vi "Test_Impression_Etiquette_Carton.vi"() -> ()   [LabVIEW 2020]
uses:
  Modules/Fonction Standard/Fichier ou dossier/Cluster des Chemins.ctl
  Flatprop/Flatprop - Standard/XML/Control/PP Param_3.ctl
panel:
  in  "DIVISION":enum16{"FLATPROP", "MEDIC"}(ring)
  in  "Pieces/carton":u16=25
  in  "Paramètres Produit (PP)":T1={"Numéro T121"="", "Créateur"="", "Date de création"="", "Date de modification"="", "indice produit"="03", "Code Barre fixe"="11210574", "Affiche n° Client [Oui/Non]"="Oui", "Fichier PTV"="", "Nbr de valves / Cartons"="25", "Mélange des lots posiible [Oui/Non] "="Non", "Affiche code barre client [Oui/Non]"="Oui", "Fichier PP valve sur embase"="", "Valve Direct/Compensée [D/C]"="D"} caption="Paramètres produit"
  in  "DATA cmde":T2={"n°article FAS"="12-216C-04521 EQIFIL 417mA 14.4ohm", "n° cmde FAS"="03838/08-01.07.01", "quantité cmde"="100", "ID LIG cmde"="966584", "n° cmde client"="CF-08-0253/2", "nom client"="EMS Electro Medical System", "n° article client"="EL-360", "indice revision client"="03", "société de facturation"="FAS Medic", "langue a utiliser"="FR"}
  in  "error in (no error)":errorcluster caption="entrée d'erreur (pas d'erreur)"
  out "error out":errorcluster caption="sortie d'erreur"
  # "Positionner sur \"MEDIC\"\npour prise en compte indicateur \n\"Pieces/carton\""
  # "Ssi Division \"MEDIC\""
  # "etiquette"
  # "(Lien interchangeable)"
  # "emballage"
  # "emballage"
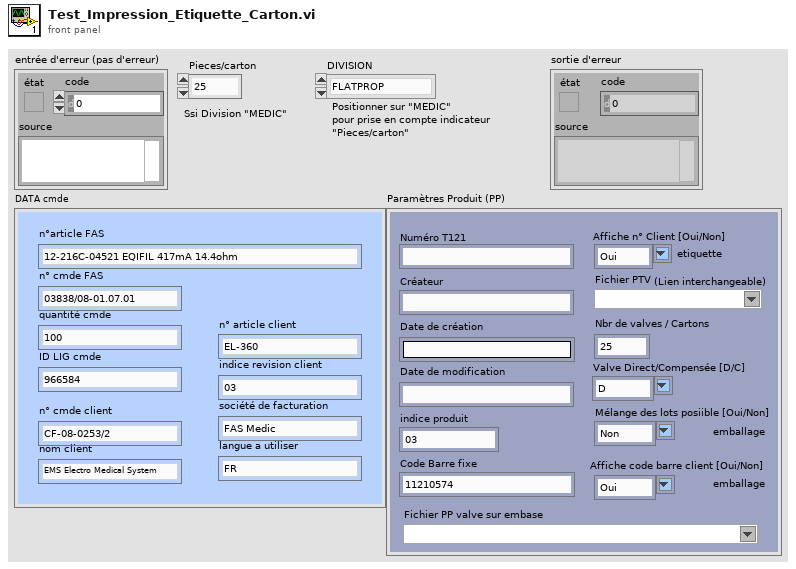
[diagram p1: front panel]
types:
  T1 = typedef "PP Param_3.ctl" = cluster{"Numéro T121":string, "Créateur":string, "Date de création":string, "Date de modification":string, "indice produit":string, "Code Barre fixe":string, "Affiche n° Client [Oui/Non]":string, "Fichier PTV":string, "Nbr de valves / Cartons":string, "Mélange des lots posiible [Oui/Non] ":string, "Affiche code barre client [Oui/Non]":string, "Fichier PP valve sur embase":string, "Valve Direct/Compensée [D/C]":string}
  T2 = typedef "DATA commande.ctl" = cluster{"n°article FAS":string, "n° cmde FAS":string, "quantité cmde":string, "ID LIG cmde":string, "n° cmde client":string, "nom client":string, "n° article client":string, "indice revision client":string, "société de facturation":string, "langue a utiliser":string}
  T3 = enum16{"Sans_imprimante", "Zebra_Medic_emballage2", "Zebra_Medic_2", "Zebra_Medic_1", "Zebra_Flat_emballage"}
  T4 = typedef "Cluster des Chemins.ctl" = cluster{" Admin-réseau ":path, " XML-Réseau":path, " Résultat tests-Réseau":path, " Archive prôbleme-Réseau":path, " Archive Test  Local":path}
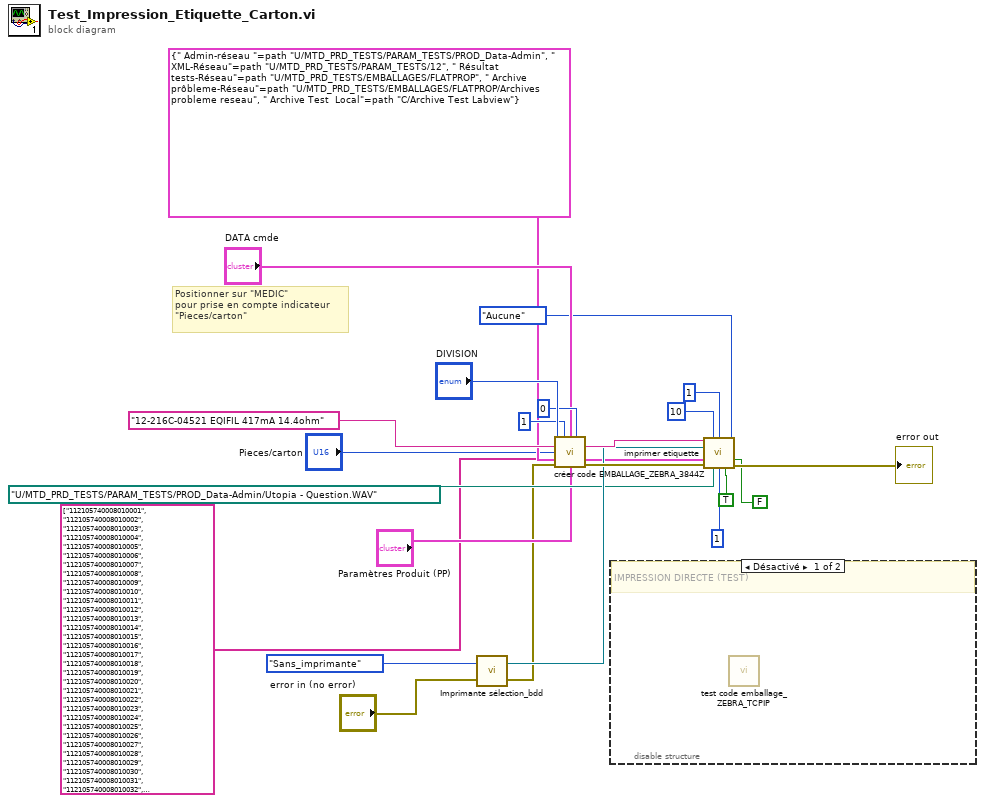
[diagram p0: block diagram]
diagram:
  # "Positionner sur \"MEDIC\"\npour prise en compte indicateur \n\"Pieces/carton\""
  n1 = call "Imprimante sélection_bdd.vi"("entrée d'erreur"="error in (no error)", "Choix imprimante"=T3."Sans_imprimante") -> ("sortie d'erreur"=w2:errorcluster, "Output ressource VISA"=w13:refnum<visa-resource-name>)
  n2 = call "créer code EMBALLAGE_ZEBRA_3844Z.vi"("DIVISION"="DIVISION", "N° carton"=u8 1, "DATA cmde"="DATA cmde", "Nb total cartons"=0, 5:"12-216C-04521 EQIFIL 417mA 14.4ohm" ("article"), 7:"Pieces/carton", "Tableau n° valves"=string[] ["112105740008010001", "112105740008010002", "112105740008010003", "112105740008010004", "112105740008010005", "112105740008010006", "112105740008010007", "112105740008010008", "112105740008010009", "112105740008010010", "112105740008010011", "112105740008010012", "112105740008010013", "112105740008010014", "112105740008010015", "112105740008010016", "112105740008010017", "112105740008010018", "112105740008010019", "112105740008010020", "112105740008010021", "112105740008010022", "112105740008010023", "112105740008010024", "112105740008010025", "112105740008010026", "112105740008010027", "112105740008010028", "112105740008010029", "112105740008010030", "112105740008010031", "112105740008010032", "112105740008010033", "112105740008010034", "112105740008010035", "112105740008010036", "112105740008010037", "112105740008010038", "112105740008010039", "112105740008010040", "112105740008010041", "112105740008010042", "112105740008010043", "112105740008010044", "112105740008010045", "112105740008010046", "112105740008010047", "112105740008010048", "112105740008010049", "112105740008010050"], "error in (no error)"=w2, 13:"Paramètres Produit (PP)") -> ("chaine  à écrire"=w22:string, "error out"=w23:errorcluster)  [unwired: 3 in, 2 out]
  n3 = disable-structure shown="Désactivé" {
    frame Disabled {
      # "IMPRESSION DIRECTE (TEST)"
      n4 = call "test code emballage_ZEBRA_TCPIP.vi"() -> ()  [unwired: 12 in]
    }
    frame Enabled {
    }
  }
  n5 = call "imprimer etiquette.vi"("chaine à écrire"=w22, "nbr de valve"=i16 10, "nbr de carton"=i16 1, "Type de liaison"=enum16{"RS232", "USB", "TCP-IP", "Aucune"}."Aucune", 5:w13, "sélecteur"=T4 {" Admin-réseau "=path "U:/MTD_PRD_TESTS/PARAM_TESTS/PROD_Data-Admin", " XML-Réseau"=path "U:/MTD_PRD_TESTS/PARAM_TESTS/12", " Résultat tests-Réseau"=path "U:/MTD_PRD_TESTS/EMBALLAGES/FLATPROP", " Archive prôbleme-Réseau"=path "U:/MTD_PRD_TESTS/EMBALLAGES/FLATPROP/Archives probleme reseau", " Archive Test  Local"=path "C:/Archive Test Labview"} ("Chemins-News"), "Cde_Interne"=FALSE, "error in"=w23, 12:path "U:/MTD_PRD_TESTS/PARAM_TESTS/PROD_Data-Admin/Utopia - Question.WAV" ("Chemin son.wav"), "Carton Numéro"=i16 1, "fin de série ?"=TRUE) -> ("error out"=→"error out":errorcluster)  [unwired: 4 in]
